vi "Recieve Request for Result.vi"(6 "Request time":timestamp, 8 "error in (no error)":errorcluster, 9 "Requestor":string, 10 "Requestee":string, 11 "Sequence Stepper in":refnum<class "Sequence Stepper.lvclass">) -> (0 "error out":errorcluster, 3 "Sequence Stepper out":refnum<class "Sequence Stepper.lvclass">)   [LabVIEW 2015, in "Sequence Stepper.lvclass"]
uses:
  Sequence Stepper.lvclass
  Mag Lab Root/Mag Lab Root.lvclass/Mag Lab Root.ctl
  Sequence Stepper.lvclass/Sequence Stepper.ctl
  <vilib>/ActorFramework/Actor/Actor.lvclass/Actor.ctl
  Mag Lab Root Messages/Recieve Request for Result Msg/Recieve Request for Result Msg.lvclass/Recieve Request for Result Msg.ctl
  <vilib>/ActorFramework/Message Enqueuer/Message Enqueuer.lvclass/Message Enqueuer.ctl
  <vilib>/ActorFramework/Message Enqueuer/Enqueue.vi
  <vilib>/ActorFramework/Message Priority Queue/Priority Enqueue.vi
  Mag Lab Root Messages/Recieve Request for Result Msg/Recieve Request for Result Msg.lvclass
  Mag Lab Root/Mag Lab Root.lvclass
  <vilib>/ActorFramework/Actor/Actor.lvclass
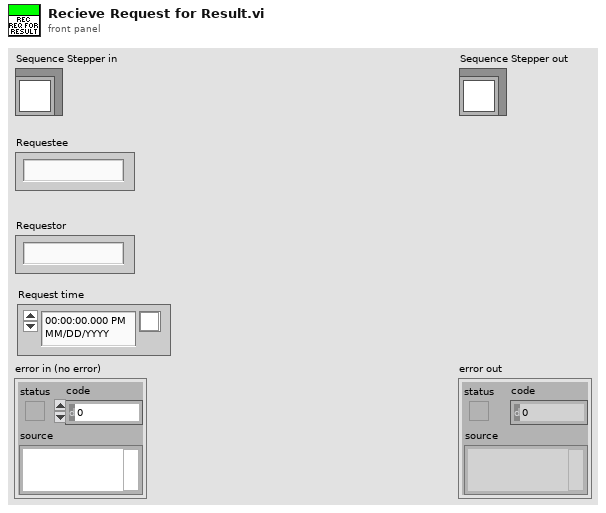
[diagram p1: front panel]
types:
  T1 = typedef "Stepper stage.ctl" = enum16{"New step", "Waiting to settle"}
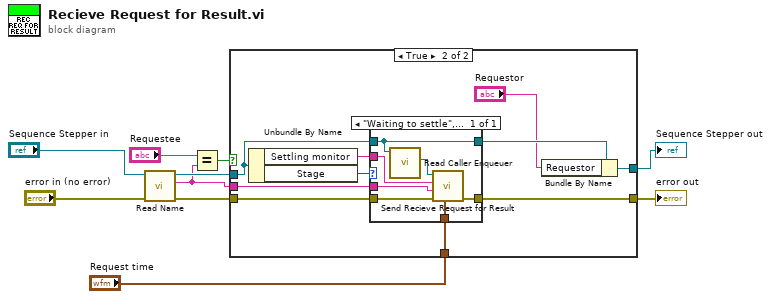
[diagram p0: block diagram]
diagram:
  n1 = call "Read Name.vi"("error in (no error)"="error in (no error)", "Mag Lab Root in"="Sequence Stepper in") -> ("error out"=w3:errorcluster, "Name"=w5:string, "Mag Lab Root out"=w6:refnum<class "Sequence Stepper.lvclass">)  [unwired: 7 in]
  n2 = Equal?(x="Requestee", y=w5) -> (x = y?=w7:bool)
  n3 = case shown="True" w7 {
    tunnel: w6 -> [w12 w19]
    tunnel: w5 -> [_ w21]
    tunnel: [w12 w16] -> w4
    tunnel: w3 -> [w11 w17]
    tunnel: [w11 w14] -> w2
    tunnel: "Request time" -> [_ w13]
    frame False {
    }
    frame True {
      n4 = Unbundle By Name(w19) -> ("Settling monitor"=w20:string, "Stage"=w22:T1)
      n5 = case shown="\"Waiting to settle\", Default" w22 {
        tunnel: w21 -> [w29]
        tunnel: w20 -> [w28]
        tunnel: w19 -> [w26]
        tunnel: [w26] -> w18
        tunnel: w17 -> [w25]
        tunnel: [w24] -> w14
        tunnel: w13 -> [w23]
        frame "Waiting to settle", Default {
          n6 = call <vilib>:"Read Caller Enqueuer.vi"("Actor"=w26) -> ("Caller Enqueuer"=w27:refnum<class "Message Enqueuer.lvclass">)  [unwired: 10 in]
          n7 = call "Send Recieve Request for Result.vi"("Request time"=w23, "error in (no error)"=w25, "Requestor"=w29, "Requestee"=w28, "Message Enqueuer"=w27) -> ("error out"=w24:errorcluster)  [unwired: 5 in, 1 out]
        }
      }
      n8 = Bundle By Name(cluster=w18, "Requestor"="Requestor") -> (w16:refnum<class "Sequence Stepper.lvclass">)
    }
  }
  "error out" <- w2
  "Sequence Stepper out" <- w4
